vi "UWBController.vi"() -> ()   [LabVIEW 2016]
doc: "UWBController sends a RESET message to the DWM over UART, then checks for a heartbeat from the DWM. When a heartbeat is found, sends a command for the DWM to broadcast its position. Then reformat the position into a global cluster variable."
uses:
  <vilib>/myRIO/Instrument Drivers/Onboard IO/UART/typedef/VISA Configuration.ctl
  <vilib>/Instr/_visa.llb/VISA Configure Serial Port (Instr).vi
  GlobalVI.vi
  <vilib>/myRIO/Express VI/Onboard IO/UART/UART Express VI.xnode
  <vilib>/regexp/Match Regular Expression.xnode
  <vilib>/myRIO/Instrument Drivers/Onboard IO/UART/UART.lvlib
panel:
  out "System ON":bool
  out "Receiving":bool
  out "Transmitting":bool
  out "Resetting...":bool
  out "X":dbl
  out "Y":dbl
  out "Z":dbl
  out "MSGFound":bool
  out "offset past match\n(-1 = no match)":i32
  out "error out OUTPUT 2":errorcluster
  in  "error in OUTPUT 2":errorcluster
  out "UART Reset Buffer":string
  out "error out INPUT":errorcluster
  in  "error in INPUT":errorcluster
  # "DWM SYSTEM"
  # "UART OUTPUT"
  # "DEBUG"
  # "COORDINATES"
  # "INPUT ERROR"
  # "OUTPUT ERROR"
  # "Input ASCII Codes\n--------------------\nlep - 108, 101, 112\nlec - 108, 101, 99\n\ncr - 13"
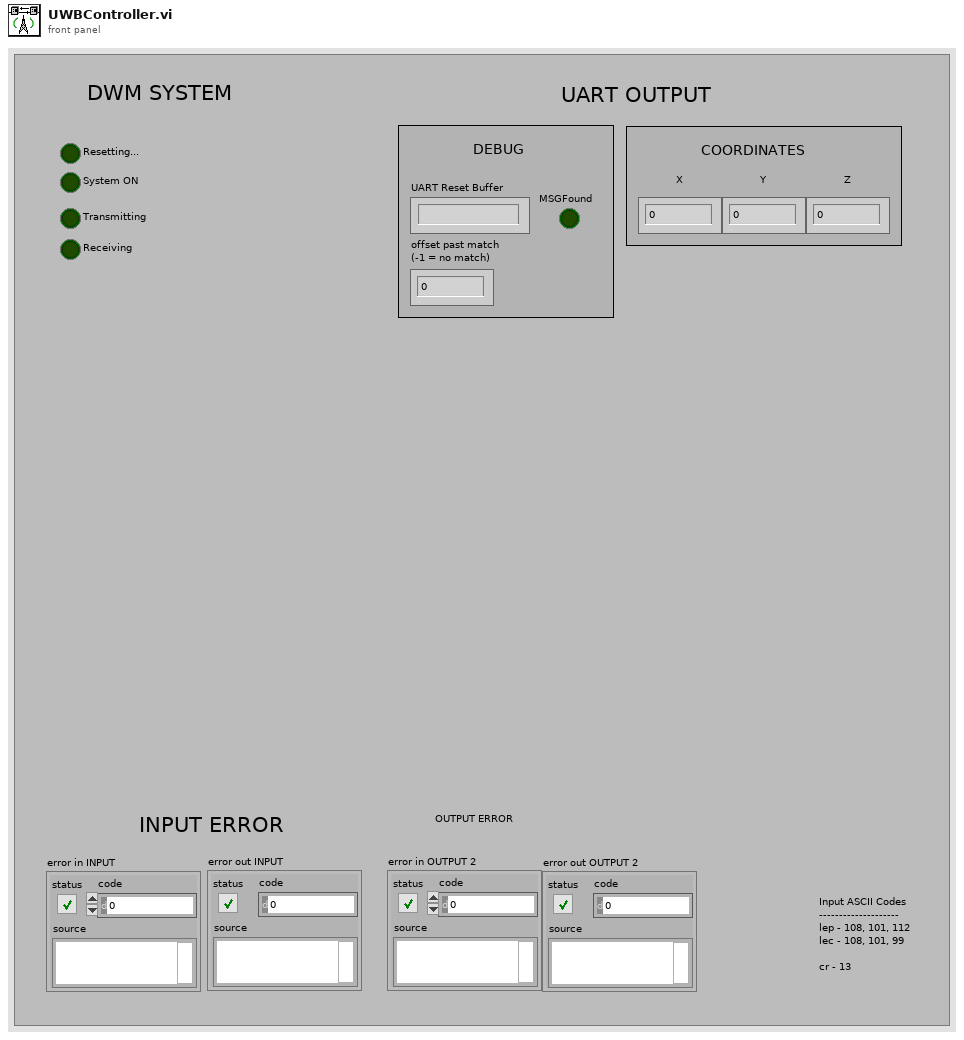
[diagram p1: front panel]
types:
  T1 = typedef "UART.lvlib/VISA Configuration.ctl" = cluster{"baud rate (9600)":u32, "data bits (8)":u16, "parity (0:none)":enum16{"None", "Odd", "Even", "Mark", "Space"}, "stop bits (10: 1 bit)":u16, "flow control (0:none)":u16, "termination char\n(0xA = '\\n' = LF) ":u8, "Enable Termination\nChar (T)":bool, "timeout (10sec)":u32}
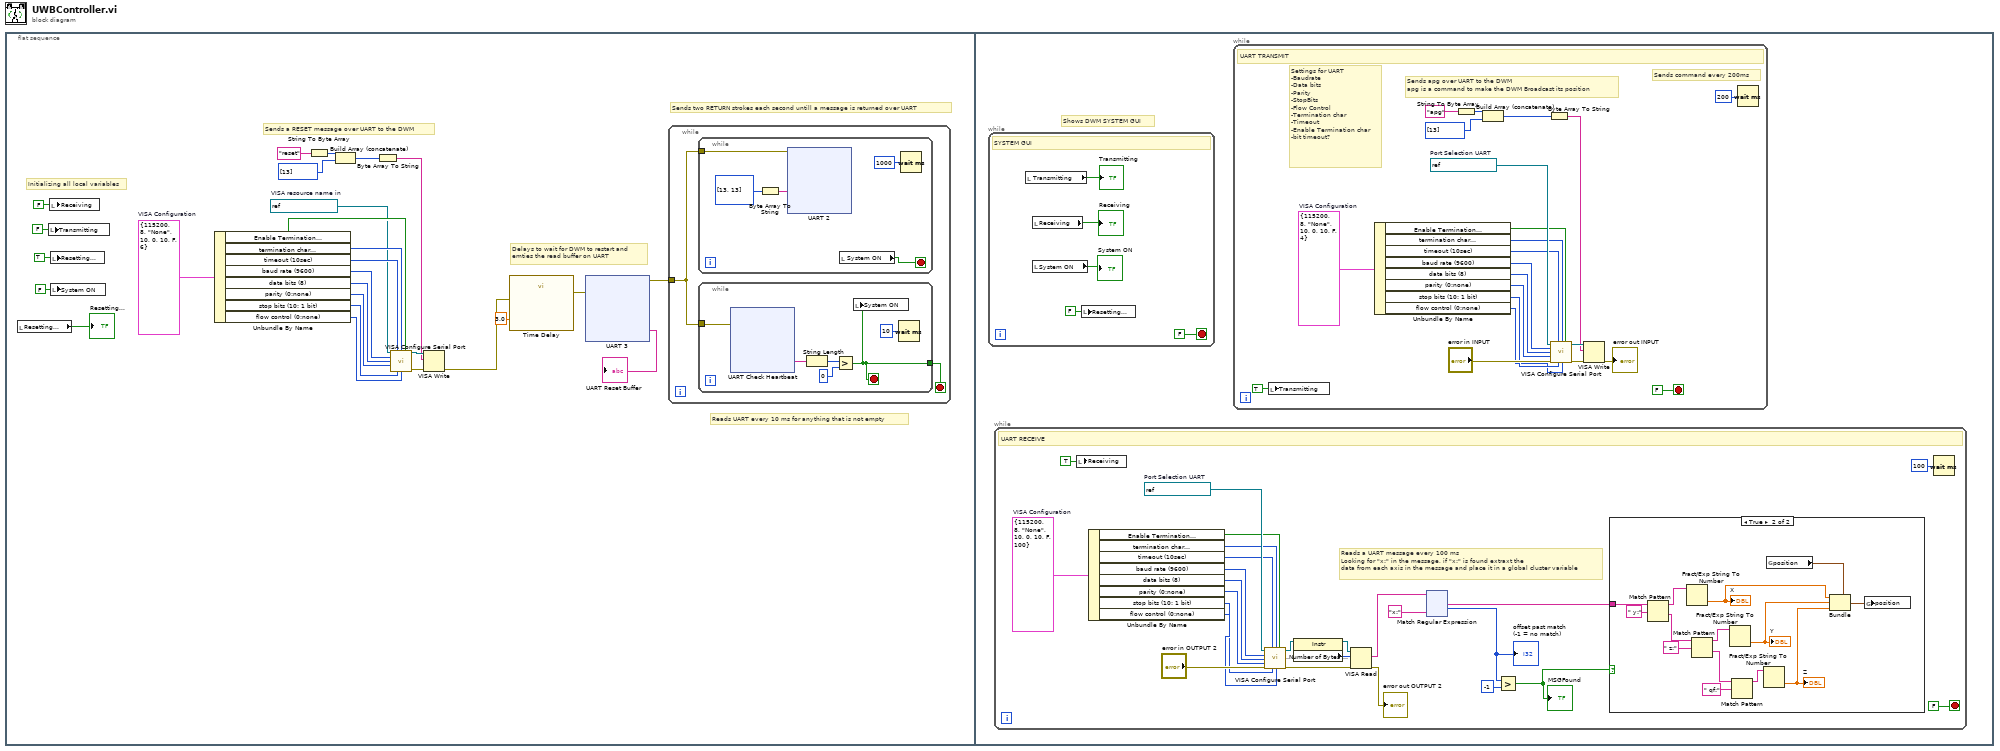
[diagram p0: block diagram]
diagram:
  n1 = flat-sequence {
    frame #0 {
      w13 = T1 {"baud rate (9600)"=115200, "data bits (8)"=8, "parity (0:none)"=enum."None", "stop bits (10: 1 bit)"=10, "flow control (0:none)"=0, "termination char\n(0xA = '\\n' = LF) "=10, "Enable Termination\nChar (T)"=FALSE, "timeout (10sec)"=6}  # VISA Configuration
      w12 = refnum<visa-resource-name> "ASRL2::INSTR"  # VISA resource name in
      # "Reads UART every 10 ms for anything that is not empty"
      # "Sends two RETURN strokes each second untill a message is returned over UART"
      # "Delays to wait for DWM to restart and \nemties the read buffer on UART"
      # "Sends a RESET message over UART to the DWM"
      # "Initializing all local variables"
      n2 = local read "Resetting..."() -> (→"Resetting...":bool)
      n3 = local write "Transmitting"(FALSE ("Transmitting")) -> ()
      n4 = local write "Receiving"(FALSE ("Receiving")) -> ()
      n5 = local write "Resetting..."(TRUE ("Resetting...")) -> ()
      n6 = local write "System ON"(FALSE ("System On")) -> ()
      n7 = Unbundle By Name(w13) -> ("Enable Termination\nChar (T)"=w16:bool, "termination char\n(0xA = '\\n' = LF)"=w17:u8, "timeout (10sec)"=w18:u32, "baud rate (9600)"=w23:u32, "data bits (8)"=w22:u16, "parity (0:none)"=w21:enum16{"None", "Odd", "Even", "Mark", "Space"}, "stop bits (10: 1 bit)"=w20:u16, "flow control (0:none)"=w19:u16)
      n8 = String To Byte Array(string="reset") -> (unsigned byte array=w8:u8[])
      n9 = Build Array (concatenate)(w8, i32[] [13]) -> (w7:i32[])
      n10 = Byte Array To String(unsigned byte array=w7) -> (string=w6:string)
      n11 = call-poly "VISA Configure Serial Port"("VISA resource name"=w12, "timeout (10sec)"=w18, "termination char\n(0xA = '\\n' = LF)"=w17, "Enable Termination\nChar (T)"=w16, "baud rate (9600)"=w23, "data bits (8)"=w22, "parity (0:none)"=w21, "stop bits (10: 1 bit)"=w20, "flow control (0:none)"=w19) -> ("VISA resource name out"=w14:refnum<visa-resource-name>, "error out"=w15:errorcluster)  [unwired: 5 in]
      n12 = VISA Write(VISA resource name=w14, write buffer=w6, error in (no error)=w15) -> (error out=w11:errorcluster)  [unwired: 2 out]
      n13 = call "Time Delay"("error in (no error)"=w11, "Delay Time (s)"=3.0) -> ("error out"=w25:errorcluster)  [unwired: 9 in]
      n14 = xnode "UART 3"("error in (no error)"=w25) -> ("Characters Read"=→"UART Reset Buffer":string, "error out"=w24:errorcluster)
      n15 = while {
        tunnel: w24 -> [w45]
        stop <- w46 stop-if-true
        n16 = while {
          tunnel: w45 -> [w47]
          stop <- w49 stop-if-true
          n17 = Byte Array To String(unsigned byte array=u8[] [13, 13]) -> (string=w51:string)
          n18 = xnode "UART 2"("Characters to Write"=w51, "error in (no error)"=w47) -> ()  [unwired: 2 out]
          n19 = local read "System ON"() -> (w49:bool)
          n20 = Wait (ms)(milliseconds to wait=u32 1000) -> ()  [unwired: 1 out]
        }
        n21 = while {
          tunnel: [w68] -> w46
          tunnel: w45 -> [w69]
          stop <- w68 stop-if-true
          n22 = xnode "UART Check Heartbeat"("error in (no error)"=w69) -> ("Characters Read"=w73:string)  [unwired: 1 out]
          n23 = String Length(string=w73) -> (length=w72:i32)
          n24 = Greater?(x=w72, y=0) -> (0:w68:bool)
          n25 = local write "System ON"(w68) -> ()
          n26 = Wait (ms)(milliseconds to wait=u32 10) -> ()  [unwired: 1 out]
        }
      }
    }
    frame #1 {
      # "Shows DWM SYSTEM GUI"
      n27 = while {
        stop <- FALSE stop-if-true
        # "SYSTEM GUI"
        n28 = local read "Transmitting"() -> (→"Transmitting":bool)
        n29 = local read "Receiving"() -> (→"Receiving":bool)
        n30 = local read "System ON"() -> (→"System ON":bool)
        n31 = local write "Resetting..."(FALSE ("Resetting...")) -> ()
      }
      n32 = while {
        stop <- FALSE stop-if-true
        w119 = T1 {"baud rate (9600)"=115200, "data bits (8)"=8, "parity (0:none)"=enum."None", "stop bits (10: 1 bit)"=10, "flow control (0:none)"=0, "termination char\n(0xA = '\\n' = LF) "=10, "Enable Termination\nChar (T)"=FALSE, "timeout (10sec)"=100}  # VISA Configuration
        w120 = refnum<visa-resource-name> "ASRL2::INSTR"  # Port Selection UART
        # "Reads a UART message every 100 ms\nLooking for \"x:\" in the message, if \"x:\" is found extraxt the\ndata from each axis in the message and place it in a global cluster variable"
        # "UART RECEIVE"
        n33 = local write "Receiving"(TRUE ("Receiving")) -> ()
        n34 = Unbundle By Name(w119) -> ("Enable Termination\nChar (T)"=w114:bool, "termination char\n(0xA = '\\n' = LF)"=w113:u8, "timeout (10sec)"=w112:u32, "baud rate (9600)"=w107:u32, "data bits (8)"=w108:u16, "parity (0:none)"=w109:enum16{"None", "Odd", "Even", "Mark", "Space"}, "stop bits (10: 1 bit)"=w110:u16, "flow control (0:none)"=w111:u16)
        n35 = call-poly "VISA Configure Serial Port"("VISA resource name"=w120, "timeout (10sec)"=w112, "termination char\n(0xA = '\\n' = LF)"=w113, "Enable Termination\nChar (T)"=w114, "baud rate (9600)"=w107, "data bits (8)"=w108, "parity (0:none)"=w109, "error in (no error)"="error in OUTPUT 2", "stop bits (10: 1 bit)"=w110, "flow control (0:none)"=w111) -> ("VISA resource name out"=w117:refnum<visa-resource-name>, "error out"=w116:errorcluster)  [unwired: 4 in]
        n36 = property class="Instr"(reference=w117) -> (reference out=w105:refnum<visa-resource-name>, "Serial Settings:Number of Bytes at Serial Port"=w106:u32)  [unwired: 1 in, 1 out]
        n37 = VISA Read(VISA resource name=w105, byte count=w106, error in (no error)=w116) -> (read buffer=w98:string, error out=→"error out OUTPUT 2":errorcluster)  [unwired: 2 out]
        n38 = xnode "Match Regular Expression"("input string"=w98, "regular expression"="x:") -> ("after match"=w97:string, "offset past match"=w102:i32)  [unwired: 4 in, 3 out]
        "offset past match\n(-1 = no match)" <- w102
        n39 = Greater?(x=w102, y=-1) -> (0:w100:bool)
        "MSGFound" <- w100
        n40 = case shown="True" w100 {
          tunnel: w97 -> [_ w126]
          frame False {
          }
          frame True {
            n41 = Match Pattern(string=w126, regular expression=" y:") -> (before substring=w133:string, after substring=w132:string)  [unwired: 1 in, 2 out]
            n42 = Fract/Exp String To Number(string=w133) -> (number=w124:dbl)  [unwired: 3 in, 1 out]
            "X" <- w124
            n43 = Match Pattern(string=w132, regular expression=" z:") -> (before substring=w130:string, after substring=w131:string)  [unwired: 1 in, 2 out]
            n44 = Fract/Exp String To Number(string=w130) -> (number=w123:dbl)  [unwired: 3 in, 1 out]
            "Y" <- w123
            n45 = Match Pattern(string=w131, regular expression=" qf:") -> (before substring=w129:string)  [unwired: 1 in, 3 out]
            n46 = Fract/Exp String To Number(string=w129) -> (number=w122:dbl)  [unwired: 3 in, 1 out]
            "Z" <- w122
            n47 = global read "GlobalVI.vi" "position"() -> (w125:cluster{"x":dbl, "y":dbl, "z":dbl})
            n48 = Bundle(cluster=w125, "x"=w124, "y"=w123, "z"=w122) -> (w121:cluster{"x":dbl, "y":dbl, "z":dbl})
            n49 = global write "GlobalVI.vi" "position"(w121) -> ()
          }
        }
        n50 = Wait (ms)(milliseconds to wait=u32 100) -> ()  [unwired: 1 out]
      }
      n51 = while {
        stop <- FALSE stop-if-true
        w269 = T1 {"baud rate (9600)"=115200, "data bits (8)"=8, "parity (0:none)"=enum."None", "stop bits (10: 1 bit)"=10, "flow control (0:none)"=0, "termination char\n(0xA = '\\n' = LF) "=10, "Enable Termination\nChar (T)"=FALSE, "timeout (10sec)"=4}  # VISA Configuration
        w270 = refnum<visa-resource-name> "ASRL2::INSTR"  # Port Selection UART
        # "Sends command every 200ms"
        # "Sends apg over UART to the DWM\napg is a command to make the DWM Broadcast its position"
        # "Settings for UART\n-Baudrate\n-Data bits\n-Parity\n-StopBits\n-Flow Control\n-Termination char\n-Timeout\n-Enable Termination char\n-bit timeout?"
        # "UART TRANSMIT"
        n52 = local write "Transmitting"(TRUE ("Transmitting")) -> ()
        n53 = Unbundle By Name(w269) -> ("Enable Termination\nChar (T)"=w265:bool, "termination char\n(0xA = '\\n' = LF)"=w264:u8, "timeout (10sec)"=w263:u32, "baud rate (9600)"=w259:u32, "data bits (8)"=w260:u16, "parity (0:none)"=w261:enum16{"None", "Odd", "Even", "Mark", "Space"}, "stop bits (10: 1 bit)"=w262:u16, "flow control (0:none)"=w257:u16)
        n54 = String To Byte Array(string="apg") -> (unsigned byte array=w254:u8[])
        n55 = Build Array (concatenate)(w254, i32[] [13]) -> (w253:i32[])
        n56 = Byte Array To String(unsigned byte array=w253) -> (string=w258:string)
        n57 = call-poly "VISA Configure Serial Port"("VISA resource name"=w270, "timeout (10sec)"=w263, "termination char\n(0xA = '\\n' = LF)"=w264, "Enable Termination\nChar (T)"=w265, "baud rate (9600)"=w259, "data bits (8)"=w260, "parity (0:none)"=w261, "error in (no error)"="error in INPUT", "stop bits (10: 1 bit)"=w262, "flow control (0:none)"=w257) -> ("VISA resource name out"=w267:refnum<visa-resource-name>, "error out"=w266:errorcluster)  [unwired: 4 in]
        n58 = VISA Write(VISA resource name=w267, write buffer=w258, error in (no error)=w266) -> (error out=→"error out INPUT":errorcluster)  [unwired: 2 out]
        n59 = Wait (ms)(milliseconds to wait=u32 200) -> ()  [unwired: 1 out]
      }
    }
  }
